vi "QT_Info.vi"(0 "QT Ref In":T4, 5 "error in (no error)":errorcluster, 8 "Private":T1) -> (9 "Info Out":T3, 10 "CIN info":string="© Chris 94-2002, QT Fat-CIN, rev: 2549, FATQTCin.c, Oct 24 2002, 14:11:49", 11 "Codec":string[](array[string])=["Animation 'rle '", "BMP 'WRLE'", "Cinepak 'cvid'", "Component Video 'yuv2'", "DV - NTSC 'dvc '", "DV - PAL 'dvcp'", "Graphics 'smc '", "H.261 'h261'", "H.263 'h263'", "Motion JPEG A 'mjpa'", "Motion JPEG B 'mjpb'", "None 'raw '", "Photo - JPEG 'jpeg'", "Planar RGB '8BPS'", "PNG 'png '", "Sorenson Video 'SVQ1'", "Sorenson Video 3 'SVQ3'", "TGA 'tga '", "TIFF 'tiff'", "Video 'rpza'"], 12 "QT Version":string="QuickTime v. 502 ", 14 "QT Ref Out":T4, 16 "QT Info":T5={"CIN info"="© Chris 94-2002, QT Fat-CIN, rev: 2549, FATQTCin.c, Oct 24 2002, 14:11:49", "CIN rev ID"=2549.0, "QT Version"="QuickTime v. 502 ", "QT option"=0, "Digitizers\n"=[], "Codec"=["Animation 'rle '", "BMP 'WRLE'", "Cinepak 'cvid'", "Component Video 'yuv2'", "DV - NTSC 'dvc '", "DV - PAL 'dvcp'", "Graphics 'smc '", "H.261 'h261'", "H.263 'h263'", "Motion JPEG A 'mjpa'", "Motion JPEG B 'mjpb'", "None 'raw '", "Photo - JPEG 'jpeg'", "Planar RGB '8BPS'", "PNG 'png '", "Sorenson Video 'SVQ1'", "Sorenson Video 3 'SVQ3'", "TGA 'tga '", "TIFF 'tiff'", "Video 'rpza'"], "reserved 1"=0, "reserved 2"=0} {"Digitizers"."In Flags" format="%.0b"; "Digitizers"."Out Flags" format="%.0b"; "Digitizers"."Inputs" items=["Composite", "S-Video", "RGB", "RGB Synch", "YUV", "YUV Synch", "TV Tuner", "sdiln"]; "CIN rev ID" format="%.2f"}, 19 "error out":errorcluster)   [LabVIEW 2024]
uses:
  <userlib>/ImageProcessing/QTLIB_2595_LV86/QT_Selector.ctl
  <userlib>/ImageProcessing/QTLIB_2595_LV86/QT_Digitizer.ctl
  <userlib>/ImageProcessing/QTLIB_2595_LV86/QT_Info.ctl
  <userlib>/ImageProcessing/QTLIB_2595_LV86/QT_Ref.ctl
  <userlib>/ImageProcessing/QTLIB_2595_LV86/QT_ErrInfo.ctl
  <userlib>/ImageProcessing/QTLIB_2595_LV86/QT_Private.ctl
panel:
  out "Codec code":string[](array[string])=["rle ", "WRLE", "cvid", "yuv2", "dvc ", "dvcp", "smc ", "h261", "h263", "mjpa", "mjpb", "raw ", "jpeg", "8BPS", "png ", "SVQ1", "SVQ3", "tga ", "tiff", "rpza"]
  out "Digitizers":T2[](array[typedef]) {"In Flags" format="%.0b"; "Out Flags" format="%.0b"; "Inputs" items=["Composite", "S-Video", "RGB", "RGB Synch", "YUV", "YUV Synch", "TV Tuner", "sdiln"]}
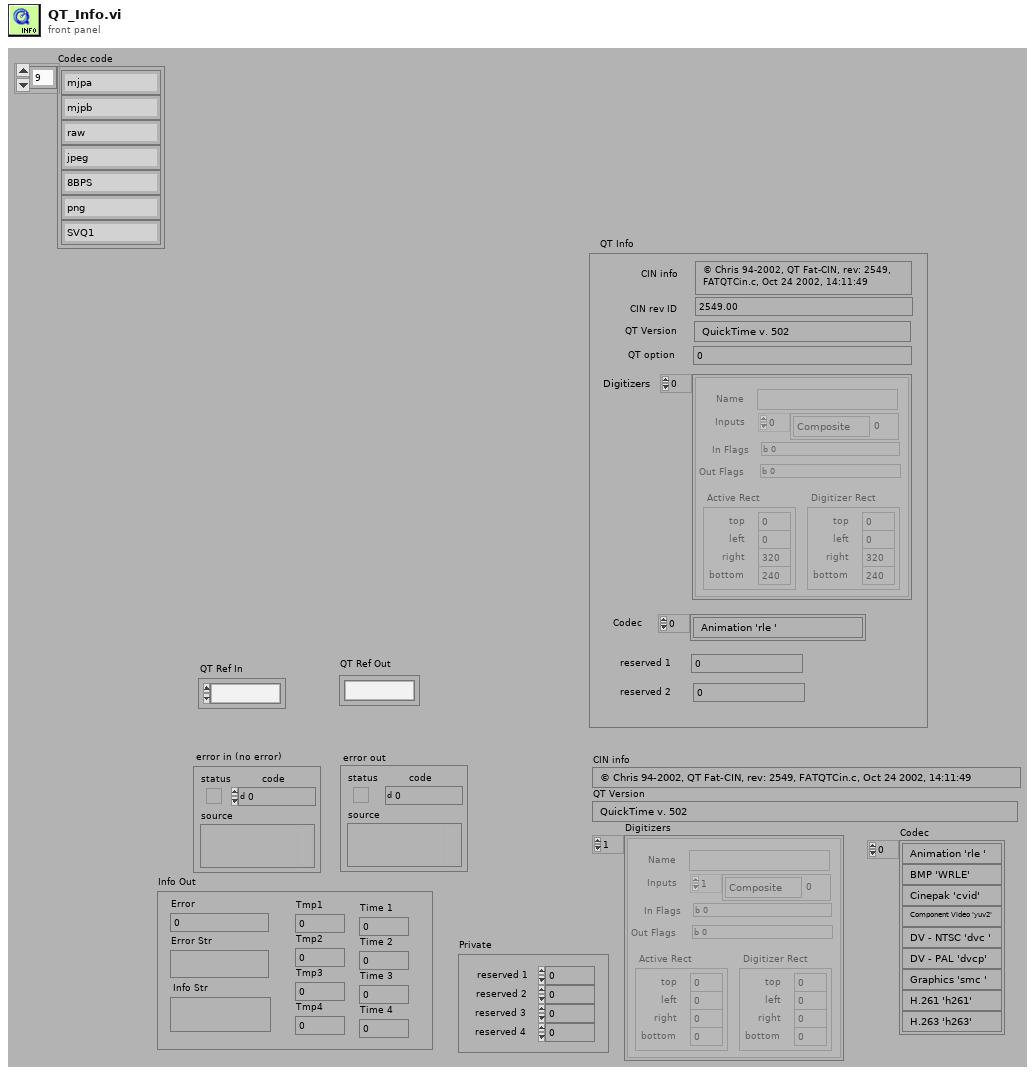
[diagram p1: front panel]
types:
  T1 = typedef "QT_Private.ctl" = cluster{"reserved 1":i32, "reserved 2":i32, "reserved 3":i32, "reserved 4":i32}
  T2 = typedef "QT_Digitizer.ctl" = cluster{"Name":string, "Inputs":i32[], "In Flags":i32, "Out Flags":i32, "Digitizer Rect":cluster{"top":i32, "left":i32, "right":i32, "bottom":i32}, "Active Rect":cluster{"top":i32, "left":i32, "right":i32, "bottom":i32}}
  T3 = typedef "QT_ErrInfo.ctl" = cluster{"Error":i32, "Error Str":string, "Info Str":string, "Tmp1":i32, "Tmp2":i32, "Tmp3":i32, "Tmp4":i32, "Time 1":i32, "Time 2":i32, "Time 3":i32, "Time 4":i32}
  T4 = typedef "QT_Ref.ctl" = refnum<k1>
  T5 = typedef "QT_Info.ctl" = cluster{"CIN info":string, "CIN rev ID":dbl, "QT Version":string, "QT option":i32, "Digitizers\n":T2[], "Codec":string[], "reserved 1":i32, "reserved 2":i32}
  T6 = typedef "QT_Selector.ctl" = enum32{"do nothing", "Get all Sources", "Get Source info", "Open Image", "Save Image to File", "Effect", "Close", "SG Grab", "Compress in Memory", "Decompress to Memory", "New Movie", "Open Movie", "Add Frame", "Get Frame", "Close Movie", "Get QT & CIN info", "SG init", "SG Close", "Open sound file", "Close sound file", "Read sound data", "Write sound data", "Import sound", "Export sound", "Add sound to movie", "Get sound from movie", "reserved", "reserved 1", "reserved 2"}
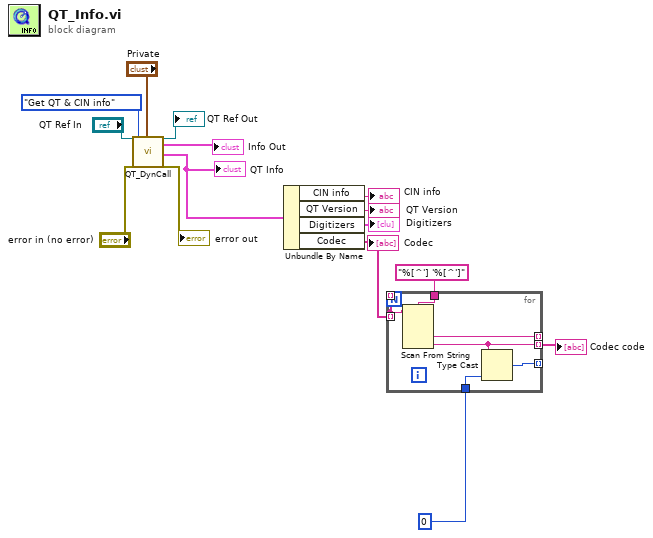
[diagram p0: block diagram]
diagram:
  n1 = call <userlib>:"QT_DynCall.vi"("QT Ref In"="QT Ref In", "error in (no error)"="error in (no error)", "Selector"=QT_Selector."Get QT & CIN info", "Private"="Private") -> ("Info Out"=→"Info Out":T3, "QT Ref Out"=→"QT Ref Out":T4, "QT Info"=w15:T5, "error out"=→"error out":errorcluster)  [unwired: 8 in, 12 out]
  "QT Info" <- w15
  n2 = Unbundle By Name(w15) -> ("CIN info"=→"CIN info":string, "QT Version"=→"QT Version":string, "Digitizers"=→"Digitizers":T2[], "Codec"=w1:string[])
  "Codec" <- w1
  n3 = for {
    tunnel: [w16] -> _ mode=indexing
    tunnel: "%[^'] '%[^']" ("format string") -> [w21]
    tunnel: [w20] -> _ mode=indexing
    tunnel: [w17] -> w2 mode=indexing
    tunnel: [w19] -> _ mode=indexing
    tunnel: u32 0 -> [w18]
    tunnel: w1 -> [w16] mode=indexing
    n4 = Scan From String(format string=w21, input string=w16) -> (output 1=w20:string, output 2=w17:string)  [unwired: 2 in, 5 out]
    n5 = Type Cast(type=w18, x=w17) -> (*(type *) &x=w19:u32)
  }
  "Codec code" <- w2
